vi "Get Request Type.vi"(8 "error in (no error)":errorcluster, 11 "GetPersistentData in":refnum<class "GetPersistentData.lvclass">) -> (0 "error out":errorcluster, 2 "Request Type":string, 3 "GetPersistentData out":refnum<class "GetPersistentData.lvclass">)   [LabVIEW 2020, in "obs-websocket.lvlib" / "GetPersistentData.lvclass"]
uses:
  GetPersistentData.lvclass
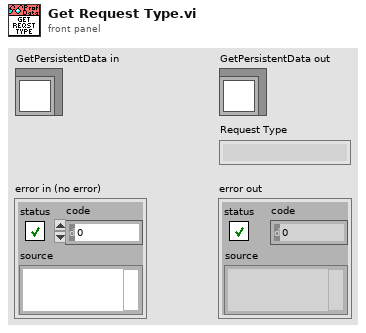
[diagram p1: front panel]
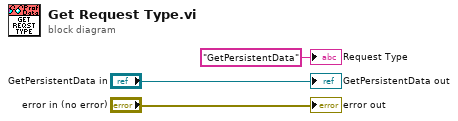
[diagram p0: block diagram]
diagram:
  "error out" <- "error in (no error)"
  "GetPersistentData out" <- "GetPersistentData in"
  "Request Type" <- "GetPersistentData" ("Request Type")
